vi "trace.vi"(2 "v":dbl=10.0, 3 "连接ID":refnum<k5>, 4 "z":dbl format="%#_13g", 5 "y":dbl, 6 "x":dbl, 7 "type":string(combo)="home") -> (0 "输出状态":string, 1 "连接ID输出":refnum<k5>)   [LabVIEW 2017]
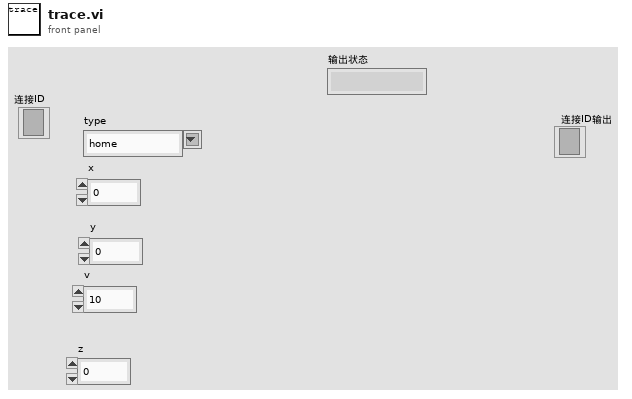
[diagram p1: front panel]
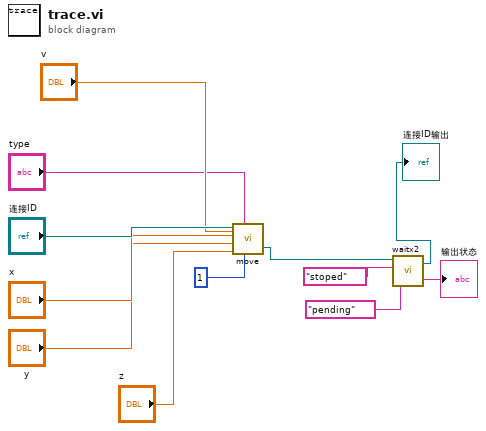
[diagram p0: block diagram]
diagram:
  n1 = call "move.vi"("v"="v", "n"=1, "String"="type", "z"="z", "y"="y", "x"="x", "连接ID"="连接ID") -> ("连接ID输出"=w10:refnum<k5>)
  n2 = call "waitx2.vi"("String Value 2"="pending", "String Value"="stoped", "连接ID"=w10) -> ("字符串"=→"输出状态":string, "连接ID 2"=→"连接ID输出":refnum<k5>)  [unwired: 1 in]
